vi "Close.vi"(8 "error in (no error)":errorcluster, 11 "Saving OO in":refnum<class "Saving OO.lvclass">) -> (0 "error out":errorcluster, 3 "Saving OO out":refnum<class "Saving OO.lvclass">)   [LabVIEW 2020, in "Saving OO.lvclass"]
uses:
  Saving OO.lvclass
  Saving OO.lvclass/Saving OO.ctl
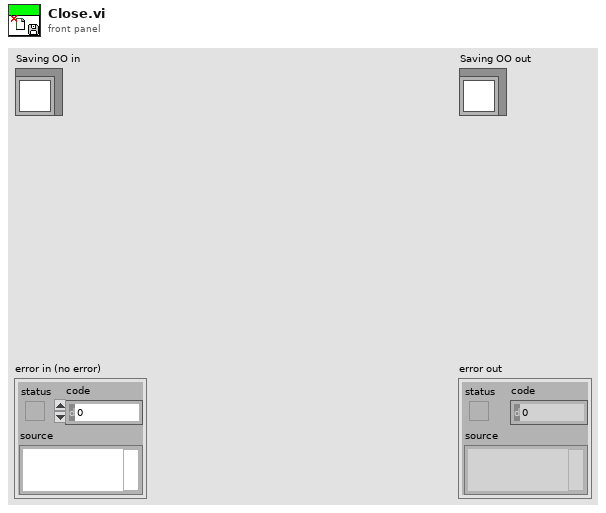
[diagram p1: front panel]
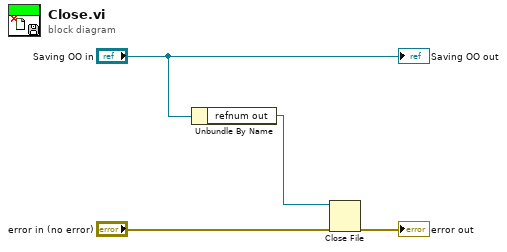
[diagram p0: block diagram]
diagram:
  n1 = Unbundle By Name("Saving OO in") -> ("refnum out"=w3:refnum<file>)
  n2 = Close File(refnum=w3, error in="error in (no error)") -> (error out=→"error out":errorcluster)  [unwired: 1 out]
  "Saving OO out" <- "Saving OO in"
